vi "TEST.vi"() -> ()   [LabVIEW 2017]
panel:
  out "error out":errorcluster
  out "Measurement":dbl
  in  "Mode clamp(only use with clamp measurement)":string(combo)="9010"
  in  "Enable Auto Range (T: Enable)":bool=TRUE
  in  "Manual Range (1.00)":dbl=1.0 format="%_3f"
  in  "Function (0: DC Voltage)":u16(ring) items=["DC Voltage", "AC Voltage", "2 - Wire Resistance", "2 -Wire Resistance low power", "4 - Wire Resistance", "4- Wire Resistance low power", "DC Current", "AC Current", "CLAMP DC", "CLAMP AC", "Frequency", "Continuity", "Diode Checking"]
  in  "VISA resource name":refnum<visa-resource-name>
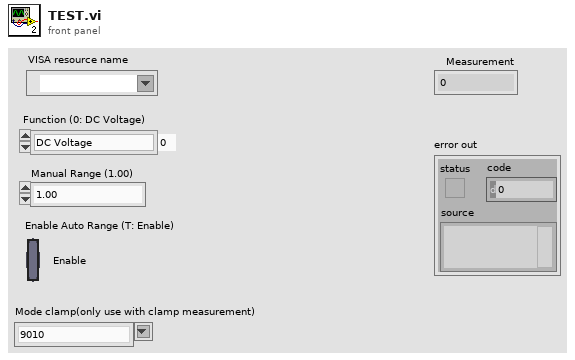
[diagram p1: front panel]
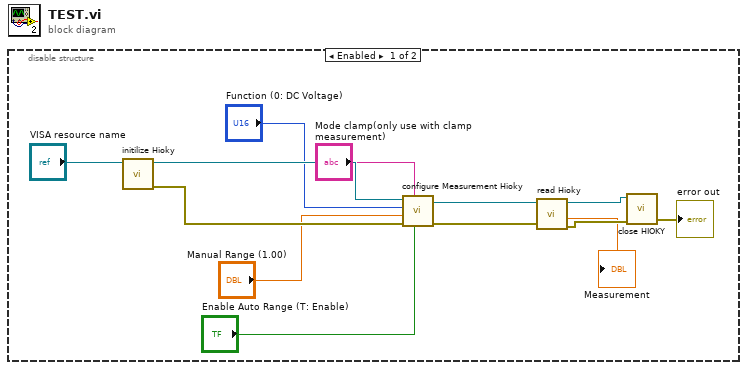
[diagram p0: block diagram]
diagram:
  n1 = disable-structure shown="Enabled" {
    frame Enabled {
      n2 = call "initilize Hioky.vi"("VISA resource name"="VISA resource name") -> ("error out"=w11:errorcluster, "VISA resource name out"=w12:refnum<visa-resource-name>)  [unwired: 9 in]
      n3 = call "configure Measurement Hioky.vi"("Enable Auto Range (T: Enable)"="Enable Auto Range (T: Enable)", "Mode clamp(only use with clamp measurement)"="Mode clamp(only use with clamp measurement)", "error in (no error)"=w11, "Manual Range (1.00)"="Manual Range (1.00)", "Function (0: DC Voltage)"="Function (0: DC Voltage)", "VISA resource name"=w12) -> ("error out"=w5:errorcluster, "VISA resource name out"=w6:refnum<visa-resource-name>)  [unwired: 4 in]
      n4 = call "read Hioky.vi"("error in (no error)"=w5, "VISA resource name"=w6) -> ("error out"=w3:errorcluster, "Measurement"=→"Measurement":dbl, "VISA resource name out"=w4:refnum<visa-resource-name>)  [unwired: 7 in]
      n5 = call "close HIOKY.vi"("error in (no error)"=w3, "VISA resource name"=w4) -> ("error out"=→"error out":errorcluster)  [unwired: 9 in]
    }
    frame Disabled {
    }
  }
